vi "data_to_xml.vi"(8 "error in (no error)":errorcluster, 11 "TTL_input in":refnum<class "TTL_input.lvclass">) -> (0 "error out":errorcluster, 2 "TTL data string":string, 3 "TTL_input out":refnum<class "TTL_input.lvclass">)   [LabVIEW 2013, in "TTL_input.lvclass"]
uses:
  TTL_input.lvclass
  TTL_input.lvclass/TTL_input.ctl
  Globals.vi
  TCP_IP/TCP_IP.lvclass
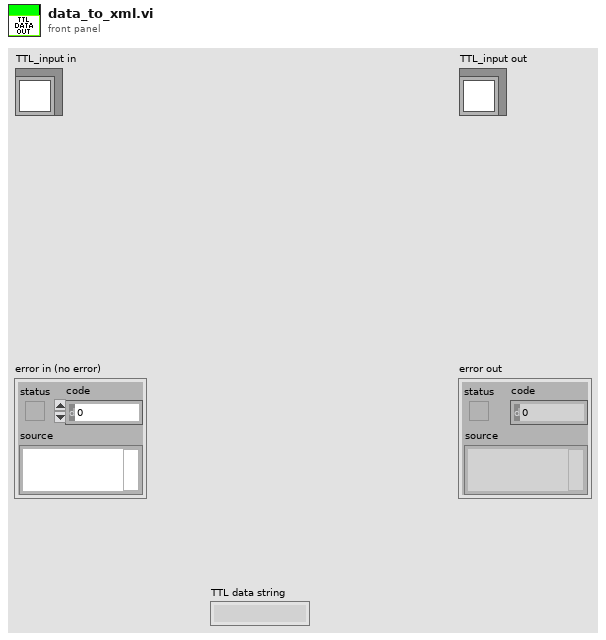
[diagram p1: front panel]
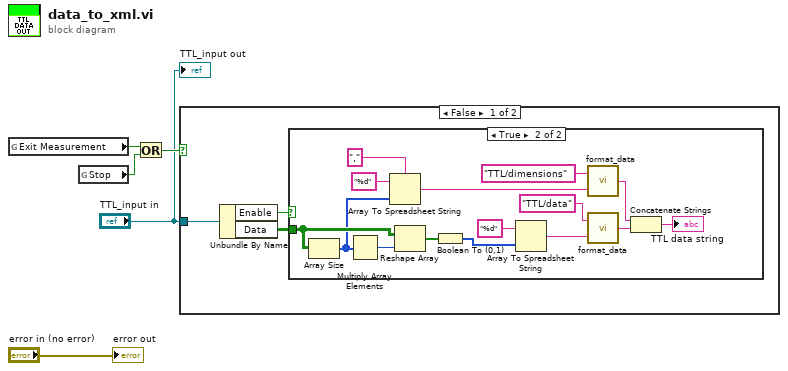
[diagram p0: block diagram]
diagram:
  n1 = global read "Globals.vi" "Exit Measurement"() -> (w5:bool)
  n2 = global read "Globals.vi" "Stop"() -> (w4:bool)
  n3 = Or(x=w5, y=w4) -> (x .or. y?=w3:bool)
  n4 = case shown="False" w3 {
    tunnel: "TTL_input in" -> [w8 _]
    frame False {
      n5 = Unbundle By Name(w8) -> ("Enable"=w7:bool, "Data"=w6:bool[][])
      n6 = case shown="True" w7 {
        tunnel: w6 -> [_ w20]
        frame False {
        }
        frame True {
          n7 = Array Size(array=w20) -> (size(s)=w19:i32[])
          n8 = Multiply Array Elements(1:w19) -> (0:w21:i32)
          n9 = Array To Spreadsheet String(delimiter (Tab)=",", array=w19, 3:"%d" ("format string")) -> (spreadsheet string=w13:string)
          n10 = Reshape Array(w20, w21) -> (w16:bool[])
          n11 = Boolean To (0,1)(Boolean=w16) -> (0, 1=w15:i16[])
          n12 = Array To Spreadsheet String(array=w15, 3:"%d" ("format string")) -> (spreadsheet string=w12:string)  [unwired: 1 in]
          n13 = call "format_data.vi"("data"=w13, "name"="TTL/dimensions") -> ("concatenated string"=w10:string)
          n14 = call "format_data.vi"("data"=w12, "name"="TTL/data") -> ("concatenated string"=w9:string)
          n15 = Concatenate Strings(w10, w9) -> (→"TTL data string":string)
        }
      }
    }
    frame True {
    }
  }
  "error out" <- "error in (no error)"
  "TTL_input out" <- "TTL_input in"
